vi "Disconnect XNodes.vi"() -> ()   [LabVIEW 2011]
panel:
  in  "target app":refnum<vi>
  in  "error out 2":errorcluster
  in  "VI Names":string[](array[string])
  out "error out":errorcluster
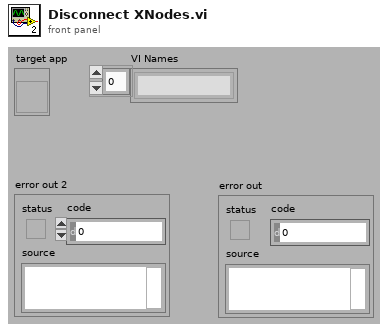
[diagram p1: front panel]
types:
  T1 = enum32{"invalid lock state", "Not Locked", "Locked (No Password)", "Password-protected"}
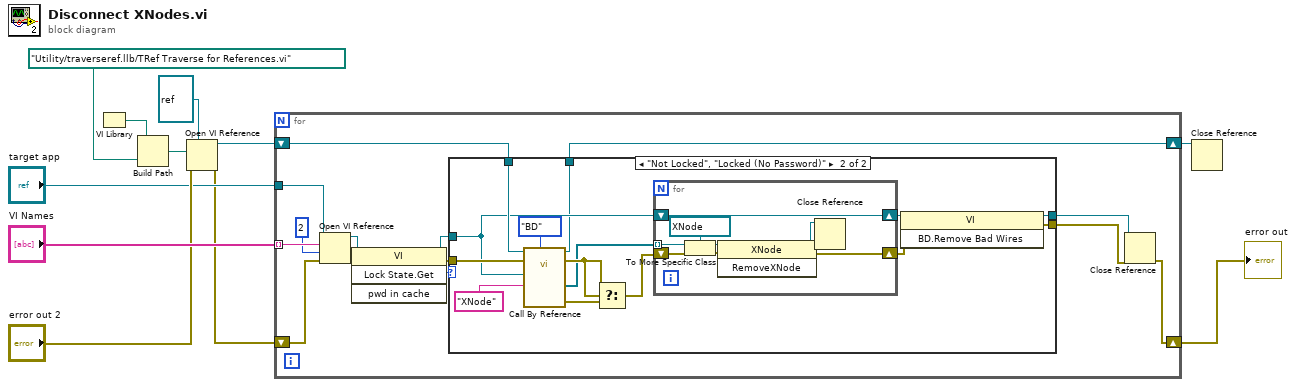
[diagram p0: block diagram]
diagram:
  n1 = VI Library() -> (path=w2:path)
  n2 = Build Path(base path=w2, name or relative path=path "Utility/traverseref.llb/TRef Traverse for References.vi" ("vi path")) -> (appended path=w4:path)
  n3 = Open VI Reference(type specifier VI Refnum (for type only)=refnum<vi> refnum, vi path=w4, error in (no error)="error out 2") -> (vi reference=w5:refnum<vi>, error out=w6:errorcluster)  [unwired: 3 in]
  n4 = for {
    tunnel: "VI Names" -> [w25] mode=indexing
    shift-right: [w23] -> w11
    shift-left: w6 -> [w24]
    shift-right: [w18] -> w7
    shift-left: w5 -> [w19]
    tunnel: "target app" -> [w17]
    n5 = Open VI Reference(application reference (local)=w17, vi path=w25, options=2, error in (no error)=w24) -> (vi reference=w16:refnum<vi>, error out=w14:errorcluster)  [unwired: 2 in]
    n6 = invoke class="VI" method="Lock State.Get"(reference=w16, error in=w14) -> (reference out=w15:refnum<vi>, error out=w13:errorcluster, "Get Lock State"=w12:T1)  [unwired: 2 in, 1 out]
    n7 = case shown="\"Not Locked\", \"Locked (No Password)\"" w12 {
      tunnel: [w27 w41] -> w21
      tunnel: [w26 w39] -> w20
      tunnel: w19 -> [w28 w38]
      tunnel: w13 -> [w26 w37]
      tunnel: w15 -> [w27 w30]
      tunnel: [w28 w29] -> w18
      frame Default {
      }
      frame "Not Locked", "Locked (No Password)" {
        n8 = call-by-ref "?"(reference=w38, error in=w37, "Traverse Target"=enum16{"FP", "BD", "Other"}."BD", "Class Name"="XNode", "VI Refnum"=w30) -> (reference out=w29:refnum<vi>, error out=w33:errorcluster, 0:"error out"=w34:errorcluster, "References"=w31:refnum<vi>[])  [unwired: 5 in, 2 out]
        n9 = Select(t=w33, s=w33, f=w34) -> (s? t:f=w32:errorcluster)
        n10 = for {
          shift-right: [w50] -> w42
          shift-left: w30 -> [w50]
          tunnel: w31 -> [w49] mode=indexing
          shift-right: [w45] -> w40
          shift-left: w32 -> [w44]
          n11 = To More Specific Class(target class=refnum<vi> refnum ("reference"), reference=w49, error in=w44) -> (specific class reference=w47:refnum<vi>, error out=w46:errorcluster)
          n12 = invoke class="XNode" method="RemoveXNode"(reference=w47, error in=w46) -> (reference out=w43:refnum<vi>, error out=w45:errorcluster)  [unwired: 1 in, 1 out]
          n13 = Close Reference(reference=w43) -> ()  [unwired: 1 in, 1 out]
        }
        n14 = invoke class="VI" method="BD.Remove Bad Wires"(reference=w42, error in=w40) -> (reference out=w41:refnum<vi>, error out=w39:errorcluster)  [unwired: 1 in, 1 out]
      }
    }
    n15 = Close Reference(reference=w21, error in (no error)=w20) -> (error out=w23:errorcluster)
  }
  "error out" <- w11
  n16 = Close Reference(reference=w7) -> ()  [unwired: 1 in, 1 out]
